vi "process.vi"(8 "error in (no error)":errorcluster, 11 "Server in":refnum<class "Server.lvclass">) -> (0 "error out":errorcluster)   [LabVIEW 2013, in "MQTT Server.lvlib" / "Server.lvclass"]
uses:
  Server.lvclass
  <vilib>/LabVIEW Open Source Project/MQTT Connection/MQTT_Base/Base Class/MQTT_Base.lvclass
  <vilib>/LabVIEW Open Source Project/MQTT Connection/MQTT_Base/Base Class/MQTT_Base.lvclass/MQTT_Base.ctl
  Server.lvclass/Server.ctl
  ConnectionHandler/ConnectionHandler.lvclass/ConnectionHandler.ctl
  ConnectionHandler/Client Event -- cluster.ctl
  ConnectionHandler/Client Action -- enum.ctl
  ConnectionHandler/ConnectionHandler.lvclass
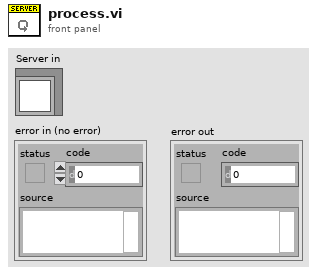
[diagram p1: front panel]
types:
  T1 = typedef "MQTT Base.lvlib/MQTT_Base.lvclass/Public Events -- cluster.ctl" = cluster{"Stop Event":refnum<user-event>, "Error Event":refnum<user-event>, "Inbound Message":refnum<user-event>}
  T2 = typedef "MQTT Server.lvlib/ConnectionHandler.lvclass/Public Events -- Cluster.ctl" = cluster{"NbConnections":refnum<user-event>, "ClientEvent":refnum<user-event>}
  T3 = typedef "MQTT Server.lvlib/ConnectionHandler.lvclass/Client Event -- cluster.ctl" = cluster{"Action":T4, "Session ID":i32}
  T4 = typedef "MQTT Server.lvlib/ConnectionHandler.lvclass/Client Action -- enum.ctl" = enum16{"Connection", "Disconnection", "Session Stored", "Session Retrieved"}
  T5 = typedef "MQTT Server.lvlib/Server.lvclass/Public Events -- cluster.ctl" = cluster{"NbConnections":refnum<user-event>, "Client Event":refnum<user-event>}
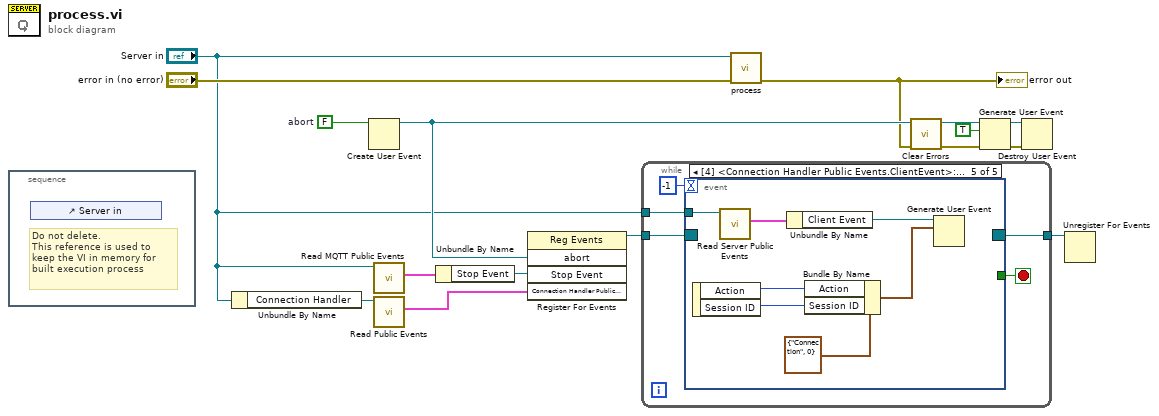
[diagram p0: block diagram]
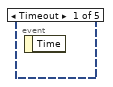
[diagram p2: hidden frame]
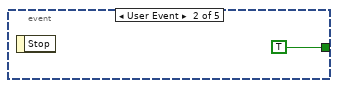
[diagram p3: hidden frame]
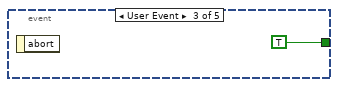
[diagram p4: hidden frame]
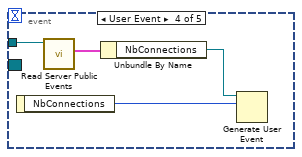
[diagram p5: hidden frame]
diagram:
  w13 = FALSE  # abort
  n1 = stacked-sequence {
    frame #0 {
      # "Do not delete.\nThis reference is used to keep the VI in memory for built execution process"
      n2 = control-ref of="Server in"() -> ()  [unwired: 1 out]
    }
  }
  n3 = Unbundle By Name("Server in") -> ("Connection Handler"=w14:refnum<class "ConnectionHandler.lvclass">)
  n4 = Create User Event(user event datatype=w13) -> (user event=w11:refnum<user-event>)  [unwired: 1 in, 1 out]
  n5 = call <vilib>:"Read MQTT Public Events.vi"("MQTT_Base in"="Server in") -> ("MQTT Public Events"=w3:T1)  [unwired: 8 in, 2 out]
  n6 = call "Read Public Events.vi"("TCPConnectionHandler in"=w14) -> ("Connection Handler Public Events"=w5:T2)  [unwired: 8 in, 2 out]
  n7 = Unbundle By Name(w3) -> ("Stop Event"=w2:refnum<user-event>)
  n8 = register-events(w11, w2, w5) -> (reference out=w12:refnum<event-registration>)  [unwired: 2 in, 1 out]
  n9 = while {
    tunnel: w12 -> [w19]
    tunnel: [w17] -> w6
    tunnel: "Server in" -> [w16]
    stop <- w18 stop-if-true
    n10 = event shown="[4] <Connection Handler Public Events.ClientEvent>: User Event" {
      selector: w19 -> [_ _ _ _ _]
      dyn-events: [_ _ _ _ _] -> w17
      timeout: -1 -> [_ _ _ _ _]
      tunnel: [_ TRUE TRUE _ _] -> w18
      tunnel: w16 -> [_ _ _ w25 w33]
      event Timeout {
        n11 = event-data() -> ()  [unwired: 1 in, 1 out]
      }
      event User Event {
        n12 = event-data() -> ()  [unwired: 1 in, 1 out]
      }
      event User Event {
        n13 = event-data() -> ()  [unwired: 1 in, 1 out]
      }
      event User Event {
        n14 = event-data() -> ("NbConnections"=w26:u32)  [unwired: 1 in]
        n15 = call "Read Server Public Events.vi"("Server in"=w25) -> ("MQTT Server.Public Events"=w24:T5)  [unwired: 8 in, 2 out]
        n16 = Unbundle By Name(w24) -> ("NbConnections"=w23:refnum<user-event>)
        n17 = Generate User Event(user event=w23, event data cluster=w26) -> ()  [unwired: 2 in, 2 out]
      }
      event User Event {
        n18 = event-data() -> ("Action"=w29:T4, "Session ID"=w28:i32)  [unwired: 1 in]
        n19 = call "Read Server Public Events.vi"("Server in"=w33) -> ("MQTT Server.Public Events"=w32:T5)  [unwired: 8 in, 2 out]
        n20 = Unbundle By Name(w32) -> ("Client Event"=w31:refnum<user-event>)
        n21 = Bundle By Name(cluster=T3 {"Action"=enum."Connection", "Session ID"=0} ("Client Event"), "Action"=w29, "Session ID"=w28) -> (w27:T3)
        n22 = Generate User Event(user event=w31, event data cluster=w27) -> ()  [unwired: 2 in, 2 out]
      }
    }
  }
  n23 = call-parent "process.vi"("error in (no error)"="error in (no error)", "MQTT_Base in"="Server in") -> ("error out"=w7:errorcluster)  [unwired: 9 in]
  "error out" <- w7
  n24 = call <vilib>:"Clear Errors.vi"("error in (no error)"=w7) -> ("error out"=w8:errorcluster)  [unwired: 6 in]
  n25 = Generate User Event(user event=w11, event data cluster=TRUE ("event data"), error in=w8) -> (user event out=w10:refnum<user-event>, error out=w9:errorcluster)  [unwired: 1 in]
  n26 = Destroy User Event(user event=w10, error in=w9) -> ()  [unwired: 1 out]
  n27 = Unregister For Events(event registration refnum=w6) -> ()  [unwired: 1 in, 1 out]
